vi "Wiimote Close.vi"(7 "Reset?":bool=TRUE, 8 "error in":errorcluster, 11 "hWiimoteHandle in":u32 format="%08x") -> (0 "error out":errorcluster)   [LabVIEW 2012, in "Wiimote.lvlib"]
uses:
  Wiimote.lvlib
  kernel32.dll
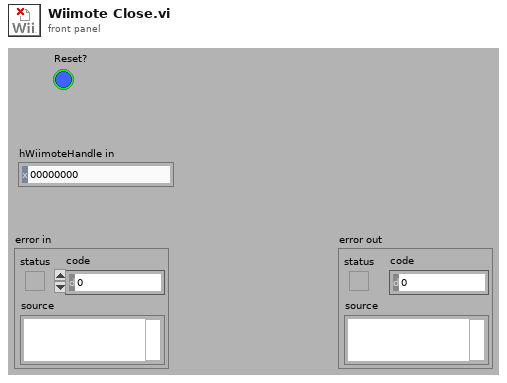
[diagram p1: front panel]
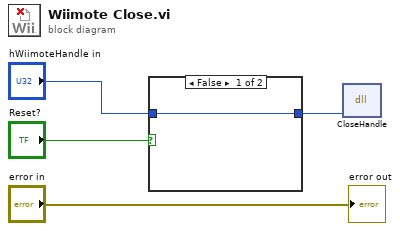
[diagram p0: block diagram]
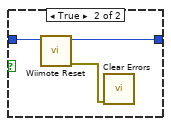
[diagram p2: hidden frame]
diagram:
  n1 = case shown="False" "Reset?" {
    tunnel: "hWiimoteHandle in" -> [w5 w8]
    tunnel: [w5 w7] -> w3
    frame False {
    }
    frame True {
      n2 = call "Wiimote Reset.vi"("hWiimoteHandle in"=w8) -> ("error out"=w6:errorcluster, "hWiimoteHandle out"=w7:u32)  [unwired: 9 in]
      n3 = call <vilib>:"Clear Errors.vi"("error in (no error)"=w6) -> ()  [unwired: 6 in, 1 out]
    }
  }
  n4 = dll-call lib="kernel32.dll" fn="CloseHandle"("hObject"=w3) -> ()  [unwired: 5 in, 2 out]
  "error out" <- "error in"
